vi "u32Scalar.vi"(4 "Numeric":u32, 5 "msg in":string) -> (2 "msg out":string)   [LabVIEW 2014]
doc: "Flattens a u32 scaler into a message"
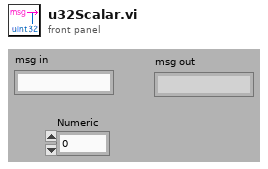
[diagram p1: front panel]
types:
  T1 = enum16{"big-endian, network order", "native, host order", "little-endian"}
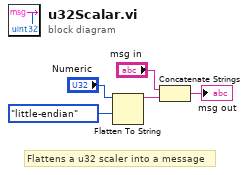
[diagram p0: block diagram]
diagram:
  # "Flattens a u32 scaler into a message"
  n1 = Flatten To String(anything="Numeric", byte order (0:big-endian, network order)=T1."little-endian") -> (data string=w3:string)  [unwired: 2 in, 2 out]
  n2 = Concatenate Strings("msg in", w3) -> (→"msg out":string)
